vi "Set Property.vi"(10 "Ctl Ref":refnum<vi>, 11 "FontUIP In":refnum<class "FontUIP.lvclass">) -> (0 "Error Out":errorcluster, 3 "FontUIP Out":refnum<class "FontUIP.lvclass">)   [LabVIEW 2016, in "FontUIP.lvclass"]
doc: "Overwrite this abstract method to implement child behavior for applying UIP private data into the VI Server Control property."
uses:
  FontUIP.lvclass
  FontUIP.lvclass/FontUIP.ctl
  <vilib>/Utility/miscctls.llb/LVRowAndColumnTypeDef.ctl
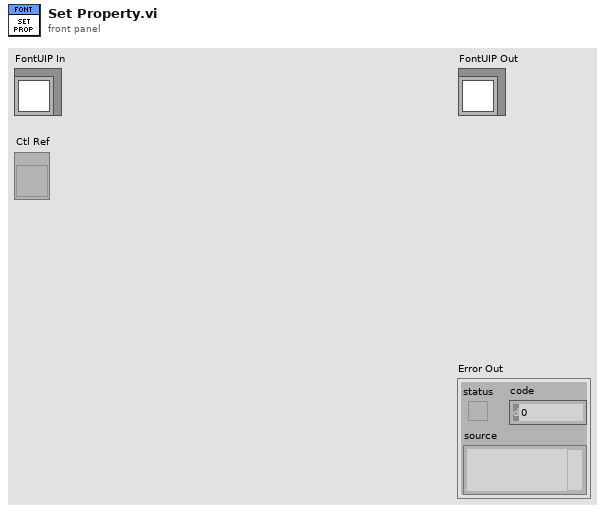
[diagram p1: front panel]
types:
  T1 = typedef "LVFontTypeDef.ctl" = cluster{"Font Name":string, "Size":u16, "Bold":bool, "Italic":bool, "Underline":bool, "Strikeout":bool, "Color":u32}
  T2 = typedef "LVRowAndColumnTypeDef.ctl" = cluster{"Row":i32, "Column":i32}
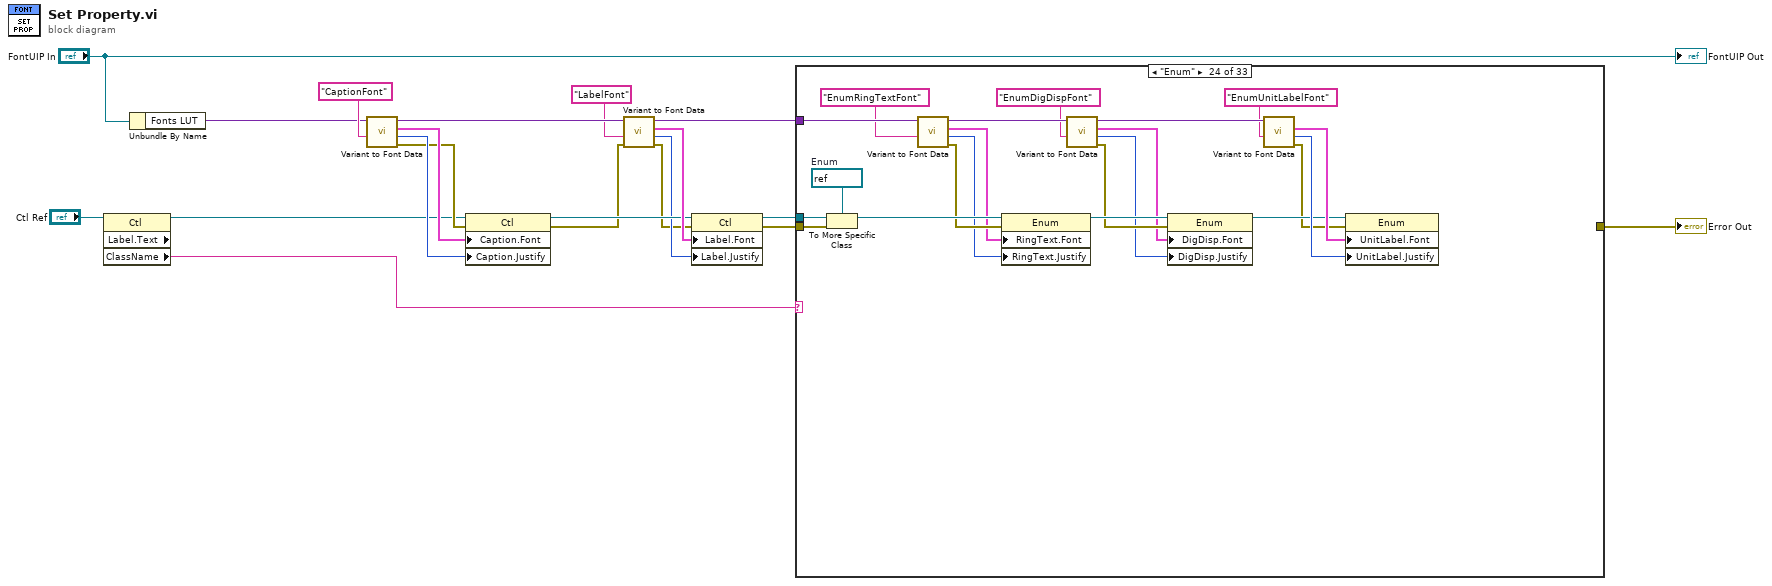
[diagram p0: block diagram]
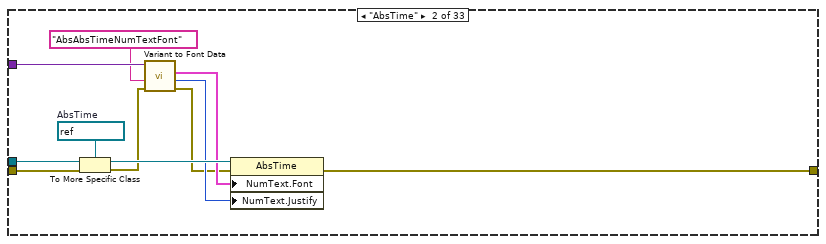
[diagram p3: hidden frame]
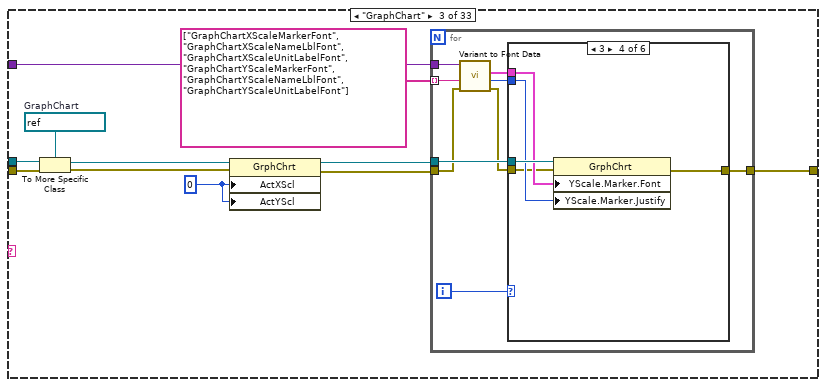
[diagram p4: hidden frame]
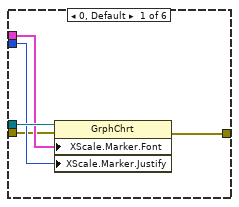
[diagram p5: hidden frame]
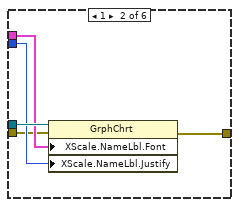
[diagram p6: hidden frame]
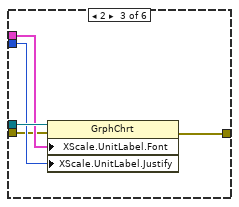
[diagram p7: hidden frame]
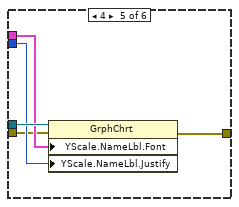
[diagram p8: hidden frame]
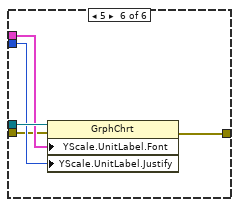
[diagram p9: hidden frame]
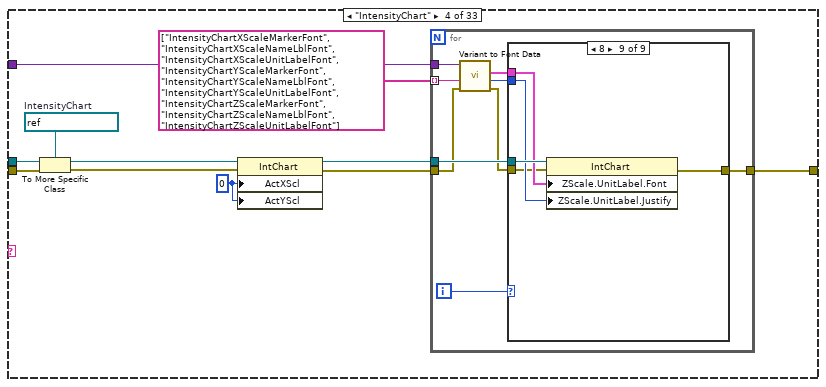
[diagram p10: hidden frame]
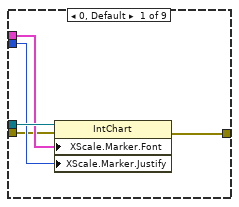
[diagram p11: hidden frame]
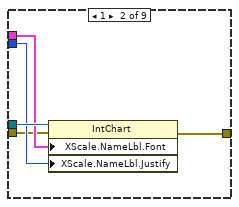
[diagram p12: hidden frame]
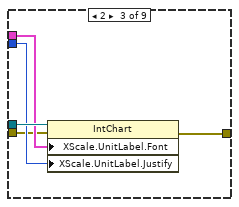
[diagram p13: hidden frame]
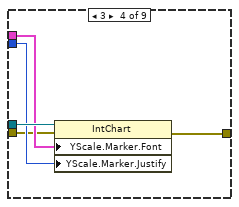
[diagram p14: hidden frame]
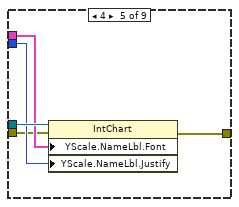
[diagram p15: hidden frame]
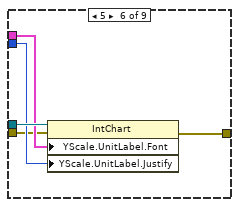
[diagram p16: hidden frame]
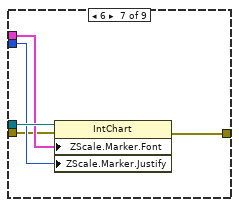
[diagram p17: hidden frame]
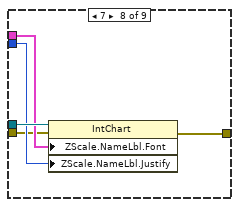
[diagram p18: hidden frame]
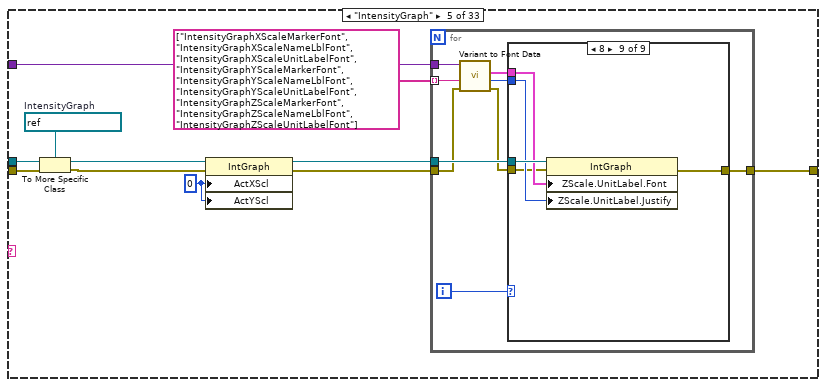
[diagram p19: hidden frame]
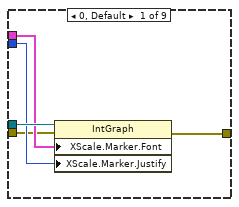
[diagram p20: hidden frame]
diagram:
  n1 = property class="Ctl" props=["Label", "Text", "ClassName"](reference="Ctl Ref") -> (reference out=w6:refnum<vi>, "ClassName"=w2:string)  [unwired: 1 in, 2 out]
  n2 = Unbundle By Name("FontUIP In") -> ("Fonts LUT"=w3:variant)
  n3 = call "Variant to Font Data.vi"("Font Key Name"="CaptionFont", "Fonts LUT in"=w3) -> ("error out"=w11:errorcluster, "Justification"=w13:enum16{"Left", "Center", "Right"}, "Font"=w12:T1, "Fonts LUT out"=w18:variant)  [unwired: 6 in]
  n4 = property class="Ctl"(reference=w6, error in=w11, "Caption.Font"=w12, "Caption.Justify"=w13) -> (reference out=w16:refnum<vi>, error out=w10:errorcluster)
  n5 = call "Variant to Font Data.vi"("error in"=w10, "Font Key Name"="LabelFont", "Fonts LUT in"=w18) -> ("error out"=w8:errorcluster, "Justification"=w9:enum16{"Left", "Center", "Right"}, "Font"=w17:T1, "Fonts LUT out"=w7:variant)  [unwired: 5 in]
  n6 = property class="Ctl"(reference=w16, error in=w8, "Label.Font"=w17, "Label.Justify"=w9) -> (reference out=w5:refnum<vi>, error out=w4:errorcluster)
  n7 = case shown="\"Enum\"" w2 {
    tunnel: w5 -> [_ w32 w42 w92 w157 w222 w272 w322 w372 w422 w473 w484 w495 w506 w517 w528 w540 w551 w563 w574 w595 w610 w631 w652 w673 w684 w701 w718 w729 w740 w751 w763 w775]
    tunnel: w7 -> [_ w27 w43 w93 w158 w223 w273 w323 w373 w423 w468 w479 w490 w501 w512 w523 w534 w546 w557 w569 w592 w607 w628 w649 w670 w679 w698 w715 w725 w735 w746 w757 w770]
    tunnel: w4 -> [w21 w31 w41 w91 w156 w221 w271 w321 w371 w421 w472 w483 w494 w505 w516 w527 w539 w550 w562 w573 w594 w609 w630 w651 w672 w683 w700 w717 w728 w739 w750 w762 w774]
    tunnel: [w21 w28 w38 w89 w153 w218 w268 w318 w368 w418 w469 w480 w491 w502 w513 w524 w535 w547 w559 w570 _ _ _ _ _ w680 _ _ w719 w736 w747 w759 w771] -> w1
    frame Default {
    }
    frame "AbsTime" {
      w29 = refnum<vi> refnum  # AbsTime
      n8 = To More Specific Class(target class=w29, reference=w32, error in=w31) -> (specific class reference=w30:refnum<vi>, error out=w23:errorcluster)
      n9 = call "Variant to Font Data.vi"("error in"=w23, "Font Key Name"="AbsAbsTimeNumTextFont", "Fonts LUT in"=w27) -> ("error out"=w22:errorcluster, "Justification"=w24:enum16{"Left", "Center", "Right"}, "Font"=w25:T1)  [unwired: 5 in, 1 out]
      n10 = property class="AbsTime"(reference=w30, error in=w22, "NumText.Font"=w25, "NumText.Justify"=w24) -> (error out=w28:errorcluster)  [unwired: 1 out]
    }
    frame "GraphChart" {
      w33 = 0 ("Active X Scale")
      w40 = refnum<vi> refnum  # GraphChart
      n11 = To More Specific Class(target class=w40, reference=w42, error in=w41) -> (specific class reference=w37:refnum<vi>, error out=w36:errorcluster)
      n12 = property class="GrphChrt"(reference=w37, error in=w36, "ActXScl"=w33, "ActYScl"=w33) -> (reference out=w35:refnum<vi>, error out=w34:errorcluster)
      n13 = for {
        tunnel: string[] ["GraphChartXScaleMarkerFont", "GraphChartXScaleNameLblFont", "GraphChartXScaleUnitLabelFont", "GraphChartYScaleMarkerFont", "GraphChartYScaleNameLblFont", "GraphChartYScaleUnitLabelFont"] -> [w51] mode=indexing
        tunnel: w43 -> [w52]
        tunnel: w35 -> [w47]
        tunnel: w34 -> [w46]
        tunnel: [w44] -> w38
        i -> [w50]
        n14 = call "Variant to Font Data.vi"("error in"=w46, "Font Key Name"=w51, "Fonts LUT in"=w52) -> ("error out"=w45:errorcluster, "Justification"=w48:enum16{"Left", "Center", "Right"}, "Font"=w49:T1)  [unwired: 5 in, 1 out]
        n15 = case shown="3" w50 {
          tunnel: w49 -> [w56 w61 w66 w71 w76 w81]
          tunnel: w48 -> [w55 w60 w65 w70 w75 w80]
          tunnel: w47 -> [w57 w62 w67 w72 w77 w82]
          tunnel: w45 -> [w54 w59 w64 w69 w74 w79]
          tunnel: [w53 w58 w63 w68 w73 w78] -> w44
          frame 0, Default {
            n16 = property class="GrphChrt"(reference=w57, error in=w54, "XScale.Marker.Font"=w56, "XScale.Marker.Justify"=w55) -> (error out=w53:errorcluster)  [unwired: 1 out]
          }
          frame 1 {
            n17 = property class="GrphChrt"(reference=w62, error in=w59, "XScale.NameLbl.Font"=w61, "XScale.NameLbl.Justify"=w60) -> (error out=w58:errorcluster)  [unwired: 1 out]
          }
          frame 2 {
            n18 = property class="GrphChrt"(reference=w67, error in=w64, "XScale.UnitLabel.Font"=w66, "XScale.UnitLabel.Justify"=w65) -> (error out=w63:errorcluster)  [unwired: 1 out]
          }
          frame 3 {
            n19 = property class="GrphChrt"(reference=w72, error in=w69, "YScale.Marker.Font"=w71, "YScale.Marker.Justify"=w70) -> (error out=w68:errorcluster)  [unwired: 1 out]
          }
          frame 4 {
            n20 = property class="GrphChrt"(reference=w77, error in=w74, "YScale.NameLbl.Font"=w76, "YScale.NameLbl.Justify"=w75) -> (error out=w73:errorcluster)  [unwired: 1 out]
          }
          frame 5 {
            n21 = property class="GrphChrt"(reference=w82, error in=w79, "YScale.UnitLabel.Font"=w81, "YScale.UnitLabel.Justify"=w80) -> (error out=w78:errorcluster)  [unwired: 1 out]
          }
        }
      }
    }
    frame "IntensityChart" {
      w83 = 0 ("Active X Scale")
      w90 = refnum<vi> refnum  # IntensityChart
      n22 = To More Specific Class(target class=w90, reference=w92, error in=w91) -> (specific class reference=w87:refnum<vi>, error out=w86:errorcluster)
      n23 = property class="IntChart"(reference=w87, error in=w86, "ActXScl"=w83, "ActYScl"=w83) -> (reference out=w85:refnum<vi>, error out=w84:errorcluster)
      n24 = for {
        tunnel: string[] ["IntensityChartXScaleMarkerFont", "IntensityChartXScaleNameLblFont", "IntensityChartXScaleUnitLabelFont", "IntensityChartYScaleMarkerFont", "IntensityChartYScaleNameLblFont", "IntensityChartYScaleUnitLabelFont", "IntensityChartZScaleMarkerFont", "IntensityChartZScaleNameLblFont", "IntensityChartZScaleUnitLabelFont"] -> [w101] mode=indexing
        tunnel: w93 -> [w102]
        tunnel: w85 -> [w97]
        tunnel: w84 -> [w96]
        tunnel: [w94] -> w89
        i -> [w100]
        n25 = call "Variant to Font Data.vi"("error in"=w96, "Font Key Name"=w101, "Fonts LUT in"=w102) -> ("error out"=w95:errorcluster, "Justification"=w98:enum16{"Left", "Center", "Right"}, "Font"=w99:T1)  [unwired: 5 in, 1 out]
        n26 = case shown="8" w100 {
          tunnel: w99 -> [w106 w111 w116 w121 w126 w131 w136 w141 w146]
          tunnel: w98 -> [w105 w110 w115 w120 w125 w130 w135 w140 w145]
          tunnel: w97 -> [w107 w112 w117 w122 w127 w132 w137 w142 w147]
          tunnel: w95 -> [w104 w109 w114 w119 w124 w129 w134 w139 w144]
          tunnel: [w103 w108 w113 w118 w123 w128 w133 w138 w143] -> w94
          frame 0, Default {
            n27 = property class="IntChart"(reference=w107, error in=w104, "XScale.Marker.Font"=w106, "XScale.Marker.Justify"=w105) -> (error out=w103:errorcluster)  [unwired: 1 out]
          }
          frame 1 {
            n28 = property class="IntChart"(reference=w112, error in=w109, "XScale.NameLbl.Font"=w111, "XScale.NameLbl.Justify"=w110) -> (error out=w108:errorcluster)  [unwired: 1 out]
          }
          frame 2 {
            n29 = property class="IntChart"(reference=w117, error in=w114, "XScale.UnitLabel.Font"=w116, "XScale.UnitLabel.Justify"=w115) -> (error out=w113:errorcluster)  [unwired: 1 out]
          }
          frame 3 {
            n30 = property class="IntChart"(reference=w122, error in=w119, "YScale.Marker.Font"=w121, "YScale.Marker.Justify"=w120) -> (error out=w118:errorcluster)  [unwired: 1 out]
          }
          frame 4 {
            n31 = property class="IntChart"(reference=w127, error in=w124, "YScale.NameLbl.Font"=w126, "YScale.NameLbl.Justify"=w125) -> (error out=w123:errorcluster)  [unwired: 1 out]
          }
          frame 5 {
            n32 = property class="IntChart"(reference=w132, error in=w129, "YScale.UnitLabel.Font"=w131, "YScale.UnitLabel.Justify"=w130) -> (error out=w128:errorcluster)  [unwired: 1 out]
          }
          frame 6 {
            n33 = property class="IntChart"(reference=w137, error in=w134, "ZScale.Marker.Font"=w136, "ZScale.Marker.Justify"=w135) -> (error out=w133:errorcluster)  [unwired: 1 out]
          }
          frame 7 {
            n34 = property class="IntChart"(reference=w142, error in=w139, "ZScale.NameLbl.Font"=w141, "ZScale.NameLbl.Justify"=w140) -> (error out=w138:errorcluster)  [unwired: 1 out]
          }
          frame 8 {
            n35 = property class="IntChart"(reference=w147, error in=w144, "ZScale.UnitLabel.Font"=w146, "ZScale.UnitLabel.Justify"=w145) -> (error out=w143:errorcluster)  [unwired: 1 out]
          }
        }
      }
    }
    frame "IntensityGraph" {
      w148 = 0 ("Active X Scale")
      w155 = refnum<vi> refnum  # IntensityGraph
      n36 = To More Specific Class(target class=w155, reference=w157, error in=w156) -> (specific class reference=w154:refnum<vi>, error out=w150:errorcluster)
      n37 = property class="IntGraph"(reference=w154, error in=w150, "ActXScl"=w148, "ActYScl"=w148) -> (reference out=w151:refnum<vi>, error out=w149:errorcluster)
      n38 = for {
        tunnel: string[] ["IntensityGraphXScaleMarkerFont", "IntensityGraphXScaleNameLblFont", "IntensityGraphXScaleUnitLabelFont", "IntensityGraphYScaleMarkerFont", "IntensityGraphYScaleNameLblFont", "IntensityGraphYScaleUnitLabelFont", "IntensityGraphZScaleMarkerFont", "IntensityGraphZScaleNameLblFont", "IntensityGraphZScaleUnitLabelFont"] -> [w166] mode=indexing
        tunnel: w158 -> [w167]
        tunnel: w151 -> [w162]
        tunnel: w149 -> [w161]
        tunnel: [w159] -> w153
        i -> [w165]
        n39 = call "Variant to Font Data.vi"("error in"=w161, "Font Key Name"=w166, "Fonts LUT in"=w167) -> ("error out"=w160:errorcluster, "Justification"=w163:enum16{"Left", "Center", "Right"}, "Font"=w164:T1)  [unwired: 5 in, 1 out]
        n40 = case shown="8" w165 {
          tunnel: w164 -> [w171 w176 w181 w186 w191 w196 w201 w206 w211]
          tunnel: w163 -> [w170 w175 w180 w185 w190 w195 w200 w205 w210]
          tunnel: w162 -> [w172 w177 w182 w187 w192 w197 w202 w207 w212]
          tunnel: w160 -> [w169 w174 w179 w184 w189 w194 w199 w204 w209]
          tunnel: [w168 w173 w178 w183 w188 w193 w198 w203 w208] -> w159
          frame 0, Default {
            n41 = property class="IntGraph"(reference=w172, error in=w169, "XScale.Marker.Font"=w171, "XScale.Marker.Justify"=w170) -> (error out=w168:errorcluster)  [unwired: 1 out]
          }
          frame 1 {
            n42 = property class="IntGraph"(reference=w177, error in=w174, "XScale.NameLbl.Font"=w176, "XScale.NameLbl.Justify"=w175) -> (error out=w173:errorcluster)  [unwired: 1 out]
          }
          frame 2 {
            n43 = property class="IntGraph"(reference=w182, error in=w179, "XScale.UnitLabel.Font"=w181, "XScale.UnitLabel.Justify"=w180) -> (error out=w178:errorcluster)  [unwired: 1 out]
          }
          frame 3 {
            n44 = property class="IntGraph"(reference=w187, error in=w184, "YScale.Marker.Font"=w186, "YScale.Marker.Justify"=w185) -> (error out=w183:errorcluster)  [unwired: 1 out]
          }
          frame 4 {
            n45 = property class="IntGraph"(reference=w192, error in=w189, "YScale.NameLbl.Font"=w191, "YScale.NameLbl.Justify"=w190) -> (error out=w188:errorcluster)  [unwired: 1 out]
          }
          frame 5 {
            n46 = property class="IntGraph"(reference=w197, error in=w194, "YScale.UnitLabel.Font"=w196, "YScale.UnitLabel.Justify"=w195) -> (error out=w193:errorcluster)  [unwired: 1 out]
          }
          frame 6 {
            n47 = property class="IntGraph"(reference=w202, error in=w199, "ZScale.Marker.Font"=w201, "ZScale.Marker.Justify"=w200) -> (error out=w198:errorcluster)  [unwired: 1 out]
          }
          frame 7 {
            n48 = property class="IntGraph"(reference=w207, error in=w204, "ZScale.NameLbl.Font"=w206, "ZScale.NameLbl.Justify"=w205) -> (error out=w203:errorcluster)  [unwired: 1 out]
          }
          frame 8 {
            n49 = property class="IntGraph"(reference=w212, error in=w209, "ZScale.UnitLabel.Font"=w211, "ZScale.UnitLabel.Justify"=w210) -> (error out=w208:errorcluster)  [unwired: 1 out]
          }
        }
      }
    }
    frame "MixedSignalGraph" {
      w213 = 0 ("Active X Scale")
      w220 = refnum<vi> refnum  # MixedSignalGraph
      n50 = To More Specific Class(target class=w220, reference=w222, error in=w221) -> (specific class reference=w219:refnum<vi>, error out=w215:errorcluster)
      n51 = property class="MixedGraph"(reference=w219, error in=w215, "ActXScl"=w213, "ActYScl"=w213) -> (reference out=w216:refnum<vi>, error out=w214:errorcluster)
      n52 = for {
        tunnel: string[] ["MixedSignalGraphXScaleMarkerFont", "MixedSignalGraphXScaleNameLblFont", "MixedSignalGraphXScaleUnitLabelFont", "MixedSignalGraphYScaleMarkerFont", "MixedSignalGraphYScaleNameLblFont", "MixedSignalGraphYScaleUnitLabelFont"] -> [w231] mode=indexing
        tunnel: w223 -> [w232]
        tunnel: w216 -> [w227]
        tunnel: w214 -> [w226]
        tunnel: [w224] -> w218
        i -> [w230]
        n53 = call "Variant to Font Data.vi"("error in"=w226, "Font Key Name"=w231, "Fonts LUT in"=w232) -> ("error out"=w225:errorcluster, "Justification"=w228:enum16{"Left", "Center", "Right"}, "Font"=w229:T1)  [unwired: 5 in, 1 out]
        n54 = case shown="0, Default" w230 {
          tunnel: w229 -> [w236 w241 w246 w251 w256 w261]
          tunnel: w228 -> [w235 w240 w245 w250 w255 w260]
          tunnel: w227 -> [w237 w242 w247 w252 w257 w262]
          tunnel: w225 -> [w234 w239 w244 w249 w254 w259]
          tunnel: [w233 w238 w243 w248 w253 w258] -> w224
          frame 0, Default {
            n55 = property class="MixedGraph"(reference=w237, error in=w234, "XScale.Marker.Font"=w236, "XScale.Marker.Justify"=w235) -> (error out=w233:errorcluster)  [unwired: 1 out]
          }
          frame 1 {
            n56 = property class="MixedGraph"(reference=w242, error in=w239, "XScale.NameLbl.Font"=w241, "XScale.NameLbl.Justify"=w240) -> (error out=w238:errorcluster)  [unwired: 1 out]
          }
          frame 2 {
            n57 = property class="MixedGraph"(reference=w247, error in=w244, "XScale.UnitLabel.Font"=w246, "XScale.UnitLabel.Justify"=w245) -> (error out=w243:errorcluster)  [unwired: 1 out]
          }
          frame 3 {
            n58 = property class="MixedGraph"(reference=w252, error in=w249, "YScale.Marker.Font"=w251, "YScale.Marker.Justify"=w250) -> (error out=w248:errorcluster)  [unwired: 1 out]
          }
          frame 4 {
            n59 = property class="MixedGraph"(reference=w257, error in=w254, "YScale.NameLbl.Font"=w256, "YScale.NameLbl.Justify"=w255) -> (error out=w253:errorcluster)  [unwired: 1 out]
          }
          frame 5 {
            n60 = property class="MixedGraph"(reference=w262, error in=w259, "YScale.UnitLabel.Font"=w261, "YScale.UnitLabel.Justify"=w260) -> (error out=w258:errorcluster)  [unwired: 1 out]
          }
        }
      }
    }
    frame "WaveformChart" {
      w263 = 0 ("Active X Scale")
      w270 = refnum<vi> refnum  # WaveformChart
      n61 = To More Specific Class(target class=w270, reference=w272, error in=w271) -> (specific class reference=w269:refnum<vi>, error out=w265:errorcluster)
      n62 = property class="WFChart"(reference=w269, error in=w265, "ActXScl"=w263, "ActYScl"=w263) -> (reference out=w266:refnum<vi>, error out=w264:errorcluster)
      n63 = for {
        tunnel: string[] ["WaveformChartXScaleMarkerFont", "WaveformChartXScaleNameLblFont", "WaveformChartXScaleUnitLabelFont", "WaveformChartYScaleMarkerFont", "WaveformChartYScaleNameLblFont", "WaveformChartYScaleUnitLabelFont"] -> [w281] mode=indexing
        tunnel: w273 -> [w282]
        tunnel: w266 -> [w277]
        tunnel: w264 -> [w276]
        tunnel: [w274] -> w268
        i -> [w280]
        n64 = call "Variant to Font Data.vi"("error in"=w276, "Font Key Name"=w281, "Fonts LUT in"=w282) -> ("error out"=w275:errorcluster, "Justification"=w278:enum16{"Left", "Center", "Right"}, "Font"=w279:T1)  [unwired: 5 in, 1 out]
        n65 = case shown="5" w280 {
          tunnel: w279 -> [w286 w291 w296 w301 w306 w311]
          tunnel: w278 -> [w285 w290 w295 w300 w305 w310]
          tunnel: w277 -> [w287 w292 w297 w302 w307 w312]
          tunnel: w275 -> [w284 w289 w294 w299 w304 w309]
          tunnel: [w283 w288 w293 w298 w303 w308] -> w274
          frame 0, Default {
            n66 = property class="WFChart"(reference=w287, error in=w284, "XScale.Marker.Font"=w286, "XScale.Marker.Justify"=w285) -> (error out=w283:errorcluster)  [unwired: 1 out]
          }
          frame 1 {
            n67 = property class="WFChart"(reference=w292, error in=w289, "XScale.NameLbl.Font"=w291, "XScale.NameLbl.Justify"=w290) -> (error out=w288:errorcluster)  [unwired: 1 out]
          }
          frame 2 {
            n68 = property class="WFChart"(reference=w297, error in=w294, "XScale.UnitLabel.Font"=w296, "XScale.UnitLabel.Justify"=w295) -> (error out=w293:errorcluster)  [unwired: 1 out]
          }
          frame 3 {
            n69 = property class="WFChart"(reference=w302, error in=w299, "YScale.Marker.Font"=w301, "YScale.Marker.Justify"=w300) -> (error out=w298:errorcluster)  [unwired: 1 out]
          }
          frame 4 {
            n70 = property class="WFChart"(reference=w307, error in=w304, "YScale.NameLbl.Font"=w306, "YScale.NameLbl.Justify"=w305) -> (error out=w303:errorcluster)  [unwired: 1 out]
          }
          frame 5 {
            n71 = property class="WFChart"(reference=w312, error in=w309, "YScale.UnitLabel.Font"=w311, "YScale.UnitLabel.Justify"=w310) -> (error out=w308:errorcluster)  [unwired: 1 out]
          }
        }
      }
    }
    frame "WaveformGraph" {
      w313 = 0 ("Active X Scale")
      w320 = refnum<vi> refnum  # WaveformGraph
      n72 = To More Specific Class(target class=w320, reference=w322, error in=w321) -> (specific class reference=w319:refnum<vi>, error out=w315:errorcluster)
      n73 = property class="WFGraph"(reference=w319, error in=w315, "ActXScl"=w313, "ActYScl"=w313) -> (reference out=w316:refnum<vi>, error out=w314:errorcluster)
      n74 = for {
        tunnel: string[] ["WaveformGraphXScaleMarkerFont", "WaveformGraphXScaleNameLblFont", "WaveformGraphXScaleUnitLabelFont", "WaveformGraphYScaleMarkerFont", "WaveformGraphYScaleNameLblFont", "WaveformGraphYScaleUnitLabelFont"] -> [w331] mode=indexing
        tunnel: w323 -> [w332]
        tunnel: w316 -> [w327]
        tunnel: w314 -> [w326]
        tunnel: [w324] -> w318
        i -> [w330]
        n75 = call "Variant to Font Data.vi"("error in"=w326, "Font Key Name"=w331, "Fonts LUT in"=w332) -> ("error out"=w325:errorcluster, "Justification"=w328:enum16{"Left", "Center", "Right"}, "Font"=w329:T1)  [unwired: 5 in, 1 out]
        n76 = case shown="4" w330 {
          tunnel: w329 -> [w336 w341 w346 w351 w356 w361]
          tunnel: w328 -> [w335 w340 w345 w350 w355 w360]
          tunnel: w327 -> [w337 w342 w347 w352 w357 w362]
          tunnel: w325 -> [w334 w339 w344 w349 w354 w359]
          tunnel: [w333 w338 w343 w348 w353 w358] -> w324
          frame 0, Default {
            n77 = property class="WFGraph"(reference=w337, error in=w334, "XScale.Marker.Font"=w336, "XScale.Marker.Justify"=w335) -> (error out=w333:errorcluster)  [unwired: 1 out]
          }
          frame 1 {
            n78 = property class="WFGraph"(reference=w342, error in=w339, "XScale.NameLbl.Font"=w341, "XScale.NameLbl.Justify"=w340) -> (error out=w338:errorcluster)  [unwired: 1 out]
          }
          frame 2 {
            n79 = property class="WFGraph"(reference=w347, error in=w344, "XScale.UnitLabel.Font"=w346, "XScale.UnitLabel.Justify"=w345) -> (error out=w343:errorcluster)  [unwired: 1 out]
          }
          frame 3 {
            n80 = property class="WFGraph"(reference=w352, error in=w349, "YScale.Marker.Font"=w351, "YScale.Marker.Justify"=w350) -> (error out=w348:errorcluster)  [unwired: 1 out]
          }
          frame 4 {
            n81 = property class="WFGraph"(reference=w357, error in=w354, "YScale.NameLbl.Font"=w356, "YScale.NameLbl.Justify"=w355) -> (error out=w353:errorcluster)  [unwired: 1 out]
          }
          frame 5 {
            n82 = property class="WFGraph"(reference=w362, error in=w359, "YScale.UnitLabel.Font"=w361, "YScale.UnitLabel.Justify"=w360) -> (error out=w358:errorcluster)  [unwired: 1 out]
          }
        }
      }
    }
    frame "DigitalGraph" {
      w363 = 0 ("Active X Scale")
      w370 = refnum<vi> refnum  # DigitalGraph
      n83 = To More Specific Class(target class=w370, reference=w372, error in=w371) -> (specific class reference=w369:refnum<vi>, error out=w365:errorcluster)
      n84 = property class="DigitalGraph"(reference=w369, error in=w365, "ActXScl"=w363, "ActYScl"=w363) -> (reference out=w366:refnum<vi>, error out=w364:errorcluster)
      n85 = for {
        tunnel: string[] ["DigitalGraphXScaleMarkerFont", "DigitalGraphXScaleNameLblFont", "DigitalGraphXScaleUnitLabelFont", "DigitalGraphYScaleMarkerFont", "DigitalGraphYScaleNameLblFont", "DigitalGraphYScaleUnitLabelFont"] -> [w381] mode=indexing
        tunnel: w373 -> [w382]
        tunnel: w366 -> [w377]
        tunnel: w364 -> [w376]
        tunnel: [w374] -> w368
        i -> [w380]
        n86 = call "Variant to Font Data.vi"("error in"=w376, "Font Key Name"=w381, "Fonts LUT in"=w382) -> ("error out"=w375:errorcluster, "Justification"=w378:enum16{"Left", "Center", "Right"}, "Font"=w379:T1)  [unwired: 5 in, 1 out]
        n87 = case shown="1" w380 {
          tunnel: w379 -> [w386 w391 w396 w401 w406 w411]
          tunnel: w378 -> [w385 w390 w395 w400 w405 w410]
          tunnel: w377 -> [w387 w392 w397 w402 w407 w412]
          tunnel: w375 -> [w384 w389 w394 w399 w404 w409]
          tunnel: [w383 w388 w393 w398 w403 w408] -> w374
          frame 0, Default {
            n88 = property class="DigitalGraph"(reference=w387, error in=w384, "XScale.Marker.Font"=w386, "XScale.Marker.Justify"=w385) -> (error out=w383:errorcluster)  [unwired: 1 out]
          }
          frame 1 {
            n89 = property class="DigitalGraph"(reference=w392, error in=w389, "XScale.NameLbl.Font"=w391, "XScale.NameLbl.Justify"=w390) -> (error out=w388:errorcluster)  [unwired: 1 out]
          }
          frame 2 {
            n90 = property class="DigitalGraph"(reference=w397, error in=w394, "XScale.UnitLabel.Font"=w396, "XScale.UnitLabel.Justify"=w395) -> (error out=w393:errorcluster)  [unwired: 1 out]
          }
          frame 3 {
            n91 = property class="DigitalGraph"(reference=w402, error in=w399, "YScale.Marker.Font"=w401, "YScale.Marker.Justify"=w400) -> (error out=w398:errorcluster)  [unwired: 1 out]
          }
          frame 4 {
            n92 = property class="DigitalGraph"(reference=w407, error in=w404, "YScale.NameLbl.Font"=w406, "YScale.NameLbl.Justify"=w405) -> (error out=w403:errorcluster)  [unwired: 1 out]
          }
          frame 5 {
            n93 = property class="DigitalGraph"(reference=w412, error in=w409, "YScale.UnitLabel.Font"=w411, "YScale.UnitLabel.Justify"=w410) -> (error out=w408:errorcluster)  [unwired: 1 out]
          }
        }
      }
    }
    frame "XYGraph" {
      w413 = 0 ("Active X Scale")
      w420 = refnum<vi> refnum  # XYGraph
      n94 = To More Specific Class(target class=w420, reference=w422, error in=w421) -> (specific class reference=w419:refnum<vi>, error out=w415:errorcluster)
      n95 = property class="XYGraph"(reference=w419, error in=w415, "ActXScl"=w413, "ActYScl"=w413) -> (reference out=w416:refnum<vi>, error out=w414:errorcluster)
      n96 = for {
        tunnel: string[] ["XYGraphXScaleMarkerFont", "XYGraphXScaleNameLblFont", "XYGraphXScaleUnitLabelFont", "XYGraphYScaleMarkerFont", "XYGraphYScaleNameLblFont", "XYGraphYScaleUnitLabelFont"] -> [w431] mode=indexing
        tunnel: w423 -> [w432]
        tunnel: w416 -> [w427]
        tunnel: w414 -> [w426]
        tunnel: [w424] -> w418
        i -> [w430]
        n97 = call "Variant to Font Data.vi"("error in"=w426, "Font Key Name"=w431, "Fonts LUT in"=w432) -> ("error out"=w425:errorcluster, "Justification"=w428:enum16{"Left", "Center", "Right"}, "Font"=w429:T1)  [unwired: 5 in, 1 out]
        n98 = case shown="1" w430 {
          tunnel: w429 -> [w436 w441 w446 w451 w456 w461]
          tunnel: w428 -> [w435 w440 w445 w450 w455 w460]
          tunnel: w427 -> [w437 w442 w447 w452 w457 w462]
          tunnel: w425 -> [w434 w439 w444 w449 w454 w459]
          tunnel: [w433 w438 w443 w448 w453 w458] -> w424
          frame 0, Default {
            n99 = property class="XYGraph"(reference=w437, error in=w434, "XScale.Marker.Font"=w436, "XScale.Marker.Justify"=w435) -> (error out=w433:errorcluster)  [unwired: 1 out]
          }
          frame 1 {
            n100 = property class="XYGraph"(reference=w442, error in=w439, "XScale.NameLbl.Font"=w441, "XScale.NameLbl.Justify"=w440) -> (error out=w438:errorcluster)  [unwired: 1 out]
          }
          frame 2 {
            n101 = property class="XYGraph"(reference=w447, error in=w444, "XScale.UnitLabel.Font"=w446, "XScale.UnitLabel.Justify"=w445) -> (error out=w443:errorcluster)  [unwired: 1 out]
          }
          frame 3 {
            n102 = property class="XYGraph"(reference=w452, error in=w449, "YScale.Marker.Font"=w451, "YScale.Marker.Justify"=w450) -> (error out=w448:errorcluster)  [unwired: 1 out]
          }
          frame 4 {
            n103 = property class="XYGraph"(reference=w457, error in=w454, "YScale.NameLbl.Font"=w456, "YScale.NameLbl.Justify"=w455) -> (error out=w453:errorcluster)  [unwired: 1 out]
          }
          frame 5 {
            n104 = property class="XYGraph"(reference=w462, error in=w459, "YScale.UnitLabel.Font"=w461, "YScale.UnitLabel.Justify"=w460) -> (error out=w458:errorcluster)  [unwired: 1 out]
          }
        }
      }
    }
    frame "Boolean" {
      w470 = refnum<vi> refnum  # Boolean
      n105 = To More Specific Class(target class=w470, reference=w473, error in=w472) -> (specific class reference=w471:refnum<vi>, error out=w467:errorcluster)
      n106 = call "Variant to Font Data.vi"("error in"=w467, "Font Key Name"="BooleanBoolTextFont", "Fonts LUT in"=w468) -> ("error out"=w466:errorcluster, "Justification"=w464:enum16{"Left", "Center", "Right"}, "Font"=w465:T1)  [unwired: 5 in, 1 out]
      n107 = property class="Bool"(reference=w471, error in=w466, "BoolText.Font"=w465, "BoolText.Justify"=w464) -> (error out=w469:errorcluster)  [unwired: 1 out]
    }
    frame "IOName" {
      w481 = refnum<vi> refnum  # IOName
      n108 = To More Specific Class(target class=w481, reference=w484, error in=w483) -> (specific class reference=w482:refnum<vi>, error out=w478:errorcluster)
      n109 = call "Variant to Font Data.vi"("error in"=w478, "Font Key Name"="IONameTextFont", "Fonts LUT in"=w479) -> ("error out"=w477:errorcluster, "Justification"=w475:enum16{"Left", "Center", "Right"}, "Font"=w476:T1)  [unwired: 5 in, 1 out]
      n110 = property class="IOName"(reference=w482, error in=w477, "Text.Font"=w476, "Text.Justify"=w475) -> (error out=w480:errorcluster)  [unwired: 1 out]
    }
    frame "DAQChannelName" {
      w492 = refnum<vi> refnum  # DAQChannelName
      n111 = To More Specific Class(target class=w492, reference=w495, error in=w494) -> (specific class reference=w493:refnum<vi>, error out=w489:errorcluster)
      n112 = call "Variant to Font Data.vi"("error in"=w489, "Font Key Name"="DAQChannelNameTextFont", "Fonts LUT in"=w490) -> ("error out"=w488:errorcluster, "Justification"=w485:enum16{"Left", "Center", "Right"}, "Font"=w486:T1)  [unwired: 5 in, 1 out]
      n113 = property class="DAQName"(reference=w493, error in=w488, "Text.Font"=w486, "Text.Justify"=w485) -> (error out=w491:errorcluster)  [unwired: 1 out]
    }
    frame "DAQmxName" {
      w503 = refnum<vi> refnum  # DAQmxName
      n114 = To More Specific Class(target class=w503, reference=w506, error in=w505) -> (specific class reference=w504:refnum<vi>, error out=w500:errorcluster)
      n115 = call "Variant to Font Data.vi"("error in"=w500, "Font Key Name"="DAQmxNameTextFont", "Fonts LUT in"=w501) -> ("error out"=w499:errorcluster, "Justification"=w497:enum16{"Left", "Center", "Right"}, "Font"=w496:T1)  [unwired: 5 in, 1 out]
      n116 = property class="DAQmxName"(reference=w504, error in=w499, "Text.Font"=w496, "Text.Justify"=w497) -> (error out=w502:errorcluster)  [unwired: 1 out]
    }
    frame "IVILogicalName" {
      w514 = refnum<vi> refnum  # IVILogicalName
      n117 = To More Specific Class(target class=w514, reference=w517, error in=w516) -> (specific class reference=w515:refnum<vi>, error out=w510:errorcluster)
      n118 = call "Variant to Font Data.vi"("error in"=w510, "Font Key Name"="IVILogicalNameTextFont", "Fonts LUT in"=w512) -> ("error out"=w509:errorcluster, "Justification"=w507:enum16{"Left", "Center", "Right"}, "Font"=w508:T1)  [unwired: 5 in, 1 out]
      n119 = property class="IVIName"(reference=w515, error in=w509, "Text.Font"=w508, "Text.Justify"=w507) -> (error out=w513:errorcluster)  [unwired: 1 out]
    }
    frame "VISAResourceName" {
      w525 = refnum<vi> refnum  # VISAResourceName
      n120 = To More Specific Class(target class=w525, reference=w528, error in=w527) -> (specific class reference=w526:refnum<vi>, error out=w522:errorcluster)
      n121 = call "Variant to Font Data.vi"("error in"=w522, "Font Key Name"="VISAResourceNameTextFont", "Fonts LUT in"=w523) -> ("error out"=w521:errorcluster, "Justification"=w519:enum16{"Left", "Center", "Right"}, "Font"=w520:T1)  [unwired: 5 in, 1 out]
      n122 = property class="VISAName"(reference=w526, error in=w521, "Text.Font"=w520, "Text.Justify"=w519) -> (error out=w524:errorcluster)  [unwired: 1 out]
    }
    frame "ListBox" {
      w537 = refnum<vi> refnum  # ListBox
      n123 = To More Specific Class(target class=w537, reference=w540, error in=w539) -> (specific class reference=w538:refnum<vi>, error out=w532:errorcluster)
      n124 = call "Variant to Font Data.vi"("error in"=w532, "Font Key Name"="ListBoxActiveRowFont", "Fonts LUT in"=w534) -> ("error out"=w531:errorcluster, "Justification"=w529:enum16{"Left", "Center", "Right"}, "Font"=w530:T1)  [unwired: 5 in, 1 out]
      n125 = property class="LstBox"(reference=w538, error in=w531, "Active Row"=-2 ("Active Row:Active Row Number"), "CellFont"=w530, "Justify"=w529) -> (error out=w535:errorcluster)  [unwired: 1 out]
    }
    frame "MixedCheckbox" {
      w548 = refnum<vi> refnum  # MixedCheckbox
      n126 = To More Specific Class(target class=w548, reference=w551, error in=w550) -> (specific class reference=w549:refnum<vi>, error out=w544:errorcluster)
      n127 = call "Variant to Font Data.vi"("error in"=w544, "Font Key Name"="MixedCheckboxTextFont", "Fonts LUT in"=w546) -> ("error out"=w543:errorcluster, "Justification"=w541:enum16{"Left", "Center", "Right"}, "Font"=w542:T1)  [unwired: 5 in, 1 out]
      n128 = property class="MixedCheckbox"(reference=w549, error in=w543, "Text.Font"=w542, "Text.Justify"=w541) -> (error out=w547:errorcluster)  [unwired: 1 out]
    }
    frame "MulticolumnListbox" {
      w560 = refnum<vi> refnum  # MulticolumnListbox
      n129 = To More Specific Class(target class=w560, reference=w563, error in=w562) -> (specific class reference=w561:refnum<vi>, error out=w555:errorcluster)
      n130 = call "Variant to Font Data.vi"("error in"=w555, "Font Key Name"="MulticolumnListboxActiveCellFont", "Fonts LUT in"=w557) -> ("error out"=w554:errorcluster, "Justification"=w552:enum16{"Left", "Center", "Right"}, "Font"=w553:T1)  [unwired: 5 in, 1 out]
      n131 = property class="MCListbox"(reference=w561, error in=w554, "ActiveCell"=T2 {"Row"=-2, "Column"=-2} ("Active Cell:Active Cell"), "CellFont"=w553, "Justify"=w552) -> (error out=w559:errorcluster)  [unwired: 1 out]
    }
    frame "Numeric" {
      w571 = refnum<vi> refnum  # Numeric
      n132 = To More Specific Class(target class=w571, reference=w574, error in=w573) -> (specific class reference=w572:refnum<vi>, error out=w568:errorcluster)
      n133 = call "Variant to Font Data.vi"("error in"=w568, "Font Key Name"="NumericUnitLabelFont", "Fonts LUT in"=w569) -> ("error out"=w567:errorcluster, "Justification"=w565:enum16{"Left", "Center", "Right"}, "Font"=w566:T1)  [unwired: 5 in, 1 out]
      n134 = property class="Num"(reference=w572, error in=w567, "UnitLabel.Font"=w566, "UnitLabel.Justify"=w565) -> (error out=w570:errorcluster)  [unwired: 1 out]
    }
    frame "ColorRamp" {
      w593 = refnum<vi> refnum  # ColorRamp
      n135 = To More Specific Class(target class=w593, reference=w595, error in=w594) -> (specific class reference=w580:refnum<vi>)  [unwired: 1 out]
      n136 = call "Variant to Font Data.vi"("Font Key Name"="ColorRampScaleMarkerFont", "Fonts LUT in"=w592) -> ("error out"=w575:errorcluster, "Justification"=w578:enum16{"Left", "Center", "Right"}, "Font"=w579:T1, "Fonts LUT out"=w591:variant)  [unwired: 6 in]
      n137 = property class="ColRmp"(reference=w580, error in=w575, "Scale.Marker.Font"=w579, "Scale.Marker.Justify"=w578) -> (reference out=w581:refnum<vi>)  [unwired: 1 out]
      n138 = call "Variant to Font Data.vi"("Font Key Name"="ColorRampDigDispFont", "Fonts LUT in"=w591) -> ("error out"=w576:errorcluster, "Justification"=w582:enum16{"Left", "Center", "Right"}, "Font"=w583:T1, "Fonts LUT out"=w590:variant)  [unwired: 6 in]
      n139 = property class="ColRmp"(reference=w581, error in=w576, "DigDisp.Font"=w583, "DigDisp.Justify"=w582) -> (reference out=w584:refnum<vi>)  [unwired: 1 out]
      n140 = call "Variant to Font Data.vi"("Font Key Name"="ColorRampUnitLabelFont", "Fonts LUT in"=w590) -> ("error out"=w577:errorcluster, "Justification"=w585:enum16{"Left", "Center", "Right"}, "Font"=w586:T1)  [unwired: 6 in, 1 out]
      n141 = property class="ColRmp"(reference=w584, error in=w577, "UnitLabel.Font"=w586, "UnitLabel.Justify"=w585) -> ()  [unwired: 2 out]
    }
    frame "Digital" {
      w608 = refnum<vi> refnum  # Digital
      n142 = To More Specific Class(target class=w608, reference=w610, error in=w609) -> (specific class reference=w600:refnum<vi>)  [unwired: 1 out]
      n143 = call "Variant to Font Data.vi"("Font Key Name"="DigitalNumTextFont", "Fonts LUT in"=w607) -> ("error out"=w597:errorcluster, "Justification"=w598:enum16{"Left", "Center", "Right"}, "Font"=w599:T1, "Fonts LUT out"=w606:variant)  [unwired: 6 in]
      n144 = property class="DigNum"(reference=w600, error in=w597, "NumText.Font"=w599, "NumText.Justify"=w598) -> (reference out=w601:refnum<vi>)  [unwired: 1 out]
      n145 = call "Variant to Font Data.vi"("Font Key Name"="DigitalUnitLabelFont", "Fonts LUT in"=w606) -> ("error out"=w596:errorcluster, "Justification"=w602:enum16{"Left", "Center", "Right"}, "Font"=w603:T1)  [unwired: 6 in, 1 out]
      n146 = property class="DigNum"(reference=w601, error in=w596, "UnitLabel.Font"=w603, "UnitLabel.Justify"=w602) -> ()  [unwired: 2 out]
    }
    frame "NamedNumeric" {
      w629 = refnum<vi> refnum  # NamedNumeric
      n147 = To More Specific Class(target class=w629, reference=w631, error in=w630) -> (specific class reference=w618:refnum<vi>)  [unwired: 1 out]
      n148 = call "Variant to Font Data.vi"("Font Key Name"="NamedNumericRingTextFont", "Fonts LUT in"=w628) -> ("error out"=w617:errorcluster, "Justification"=w615:enum16{"Left", "Center", "Right"}, "Font"=w616:T1, "Fonts LUT out"=w627:variant)  [unwired: 6 in]
      n149 = property class="NmdNum"(reference=w618, error in=w617, "RingText.Font"=w616, "RingText.Justify"=w615) -> (reference out=w619:refnum<vi>)  [unwired: 1 out]
      n150 = call "Variant to Font Data.vi"("Font Key Name"="NamedNumericDigDispFont", "Fonts LUT in"=w627) -> ("error out"=w613:errorcluster, "Justification"=w611:enum16{"Left", "Center", "Right"}, "Font"=w612:T1, "Fonts LUT out"=w626:variant)  [unwired: 6 in]
      n151 = property class="NmdNum"(reference=w619, error in=w613, "DigDisp.Font"=w612, "DigDisp.Justify"=w611) -> (reference out=w620:refnum<vi>)  [unwired: 1 out]
      n152 = call "Variant to Font Data.vi"("Font Key Name"="NamedNumericUnitLabelFont", "Fonts LUT in"=w626) -> ("error out"=w614:errorcluster, "Justification"=w621:enum16{"Left", "Center", "Right"}, "Font"=w622:T1)  [unwired: 6 in, 1 out]
      n153 = property class="NmdNum"(reference=w620, error in=w614, "UnitLabel.Font"=w622, "UnitLabel.Justify"=w621) -> ()  [unwired: 2 out]
    }
    frame "Enum" {
      w650 = refnum<vi> refnum  # Enum
      n154 = To More Specific Class(target class=w650, reference=w652, error in=w651) -> (specific class reference=w639:refnum<vi>)  [unwired: 1 out]
      n155 = call "Variant to Font Data.vi"("Font Key Name"="EnumRingTextFont", "Fonts LUT in"=w649) -> ("error out"=w638:errorcluster, "Justification"=w636:enum16{"Left", "Center", "Right"}, "Font"=w637:T1, "Fonts LUT out"=w648:variant)  [unwired: 6 in]
      n156 = property class="Enum"(reference=w639, error in=w638, "RingText.Font"=w637, "RingText.Justify"=w636) -> (reference out=w640:refnum<vi>)  [unwired: 1 out]
      n157 = call "Variant to Font Data.vi"("Font Key Name"="EnumDigDispFont", "Fonts LUT in"=w648) -> ("error out"=w634:errorcluster, "Justification"=w632:enum16{"Left", "Center", "Right"}, "Font"=w633:T1, "Fonts LUT out"=w647:variant)  [unwired: 6 in]
      n158 = property class="Enum"(reference=w640, error in=w634, "DigDisp.Font"=w633, "DigDisp.Justify"=w632) -> (reference out=w641:refnum<vi>)  [unwired: 1 out]
      n159 = call "Variant to Font Data.vi"("Font Key Name"="EnumUnitLabelFont", "Fonts LUT in"=w647) -> ("error out"=w635:errorcluster, "Justification"=w642:enum16{"Left", "Center", "Right"}, "Font"=w643:T1)  [unwired: 6 in, 1 out]
      n160 = property class="Enum"(reference=w641, error in=w635, "UnitLabel.Font"=w643, "UnitLabel.Justify"=w642) -> ()  [unwired: 2 out]
    }
    frame "Ring" {
      w671 = refnum<vi> refnum  # Ring
      n161 = To More Specific Class(target class=w671, reference=w673, error in=w672) -> (specific class reference=w660:refnum<vi>)  [unwired: 1 out]
      n162 = call "Variant to Font Data.vi"("Font Key Name"="RingRingTextFont", "Fonts LUT in"=w670) -> ("error out"=w659:errorcluster, "Justification"=w657:enum16{"Left", "Center", "Right"}, "Font"=w658:T1, "Fonts LUT out"=w669:variant)  [unwired: 6 in]
      n163 = property class="Ring"(reference=w660, error in=w659, "RingText.Font"=w658, "RingText.Justify"=w657) -> (reference out=w661:refnum<vi>)  [unwired: 1 out]
      n164 = call "Variant to Font Data.vi"("Font Key Name"="RingDigDispFont", "Fonts LUT in"=w669) -> ("error out"=w655:errorcluster, "Justification"=w653:enum16{"Left", "Center", "Right"}, "Font"=w654:T1, "Fonts LUT out"=w668:variant)  [unwired: 6 in]
      n165 = property class="Ring"(reference=w661, error in=w655, "DigDisp.Font"=w654, "DigDisp.Justify"=w653) -> (reference out=w662:refnum<vi>)  [unwired: 1 out]
      n166 = call "Variant to Font Data.vi"("Font Key Name"="RingUnitLabelFont", "Fonts LUT in"=w668) -> ("error out"=w656:errorcluster, "Justification"=w663:enum16{"Left", "Center", "Right"}, "Font"=w664:T1)  [unwired: 6 in, 1 out]
      n167 = property class="Ring"(reference=w662, error in=w656, "UnitLabel.Font"=w664, "UnitLabel.Justify"=w663) -> ()  [unwired: 2 out]
    }
    frame "NumericWithScale" {
      w681 = refnum<vi> refnum  # NumericWithScale
      n168 = To More Specific Class(target class=w681, reference=w684, error in=w683) -> (specific class reference=w682:refnum<vi>, error out=w677:errorcluster)
      n169 = call "Variant to Font Data.vi"("error in"=w677, "Font Key Name"="NumericWithScaleUnitLabelFont", "Fonts LUT in"=w679) -> ("error out"=w676:errorcluster, "Justification"=w674:enum16{"Left", "Center", "Right"}, "Font"=w675:T1)  [unwired: 5 in, 1 out]
      n170 = property class="NumWthScl"(reference=w682, error in=w676, "UnitLabel.Font"=w675, "UnitLabel.Justify"=w674) -> (error out=w680:errorcluster)  [unwired: 1 out]
    }
    frame "Knob" {
      w699 = refnum<vi> refnum  # Knob
      n171 = To More Specific Class(target class=w699, reference=w701, error in=w700) -> (specific class reference=w689:refnum<vi>, error out=w692:errorcluster)
      n172 = call "Variant to Font Data.vi"("error in"=w692, "Font Key Name"="KnobMarkerFont", "Fonts LUT in"=w698) -> ("error out"=w685:errorcluster, "Justification"=w686:enum16{"Left", "Center", "Right"}, "Font"=w687:T1, "Fonts LUT out"=w697:variant)  [unwired: 5 in]
      n173 = property class="Knob"(reference=w689, error in=w685, "Active Slider"=0, "Scale.Marker.Font"=w687, "Scale.Marker.Justify"=w686) -> (reference out=w688:refnum<vi>)  [unwired: 1 out]
      n174 = call "Variant to Font Data.vi"("Font Key Name"="KnobUnitLabelFont", "Fonts LUT in"=w697) -> ("error out"=w691:errorcluster, "Justification"=w693:enum16{"Left", "Center", "Right"}, "Font"=w694:T1)  [unwired: 6 in, 1 out]
      n175 = property class="Knob"(reference=w688, error in=w691, "UnitLabel.Font"=w694, "UnitLabel.Justify"=w693) -> ()  [unwired: 2 out]
    }
    frame "Slide" {
      w716 = refnum<vi> refnum  # Slide
      n176 = To More Specific Class(target class=w716, reference=w718, error in=w717) -> (specific class reference=w706:refnum<vi>, error out=w709:errorcluster)
      n177 = call "Variant to Font Data.vi"("error in"=w709, "Font Key Name"="SlideScaleMarkerFont", "Fonts LUT in"=w715) -> ("error out"=w702:errorcluster, "Justification"=w703:enum16{"Left", "Center", "Right"}, "Font"=w704:T1, "Fonts LUT out"=w714:variant)  [unwired: 5 in]
      n178 = property class="Slide"(reference=w706, error in=w702, "Active Slider"=0, "Scale.Marker.Font"=w704, "Scale.Marker.Justify"=w703) -> (reference out=w705:refnum<vi>)  [unwired: 1 out]
      n179 = call "Variant to Font Data.vi"("Font Key Name"="SlideUnitLabelFont", "Fonts LUT in"=w714) -> ("error out"=w708:errorcluster, "Justification"=w710:enum16{"Left", "Center", "Right"}, "Font"=w711:T1)  [unwired: 6 in, 1 out]
      n180 = property class="Slide"(reference=w705, error in=w708, "UnitLabel.Font"=w711, "UnitLabel.Justify"=w710) -> ()  [unwired: 2 out]
    }
    frame "Path" {
      w726 = refnum<vi> refnum  # Path
      n181 = To More Specific Class(target class=w726, reference=w729, error in=w728) -> (specific class reference=w727:refnum<vi>, error out=w720:errorcluster)
      n182 = call "Variant to Font Data.vi"("error in"=w720, "Font Key Name"="PathTextFont", "Fonts LUT in"=w725) -> ("error out"=w721:errorcluster, "Justification"=w722:enum16{"Left", "Center", "Right"}, "Font"=w723:T1)  [unwired: 5 in, 1 out]
      n183 = property class="Path"(reference=w727, error in=w721, "Text.Font"=w723, "Text.Justify"=w722) -> (error out=w719:errorcluster)  [unwired: 1 out]
    }
    frame "String" {
      w737 = refnum<vi> refnum  # String
      n184 = To More Specific Class(target class=w737, reference=w740, error in=w739) -> (specific class reference=w738:refnum<vi>, error out=w733:errorcluster)
      n185 = call "Variant to Font Data.vi"("error in"=w733, "Font Key Name"="StringTextFont", "Fonts LUT in"=w735) -> ("error out"=w732:errorcluster, "Justification"=w730:enum16{"Left", "Center", "Right"}, "Font"=w731:T1)  [unwired: 5 in, 1 out]
      n186 = property class="Str"(reference=w738, error in=w732, "Text.Font"=w731, "Text.Justify"=w730) -> (error out=w736:errorcluster)  [unwired: 1 out]
    }
    frame "ComboBox" {
      w748 = refnum<vi> refnum  # ComboBox
      n187 = To More Specific Class(target class=w748, reference=w751, error in=w750) -> (specific class reference=w749:refnum<vi>, error out=w744:errorcluster)
      n188 = call "Variant to Font Data.vi"("error in"=w744, "Font Key Name"="ComboBoxTextFont", "Fonts LUT in"=w746) -> ("error out"=w743:errorcluster, "Justification"=w741:enum16{"Left", "Center", "Right"}, "Font"=w742:T1)  [unwired: 5 in, 1 out]
      n189 = property class="CmbBox"(reference=w749, error in=w743, "Text.Font"=w742, "Text.Justify"=w741) -> (error out=w747:errorcluster)  [unwired: 1 out]
    }
    frame "Table" {
      w760 = refnum<vi> refnum  # Table
      n190 = To More Specific Class(target class=w760, reference=w763, error in=w762) -> (specific class reference=w761:refnum<vi>, error out=w755:errorcluster)
      n191 = call "Variant to Font Data.vi"("error in"=w755, "Font Key Name"="TableActiveCellFont", "Fonts LUT in"=w757) -> ("error out"=w754:errorcluster, "Justification"=w752:enum16{"Left", "Center", "Right"}, "Font"=w753:T1)  [unwired: 5 in, 1 out]
      n192 = property class="Tbl"(reference=w761, error in=w754, "Active Cell"=T2 {"Row"=-2, "Column"=-2} ("Active Cell:Active Cell"), "CellFont"=w753, "Justify"=w752) -> (error out=w759:errorcluster)  [unwired: 1 out]
    }
    frame "TreeControl" {
      w772 = refnum<vi> refnum  # TreeControl
      n193 = To More Specific Class(target class=w772, reference=w775, error in=w774) -> (specific class reference=w773:refnum<vi>, error out=w768:errorcluster)
      n194 = call "Variant to Font Data.vi"("error in"=w768, "Font Key Name"="TreeControlActiveColFont", "Fonts LUT in"=w770) -> ("error out"=w767:errorcluster, "Justification"=w765:enum16{"Left", "Center", "Right"}, "Font"=w766:T1)  [unwired: 5 in, 1 out]
      n195 = property class="Tree"(reference=w773, error in=w767, "ActiveColNum"=-2 ("Active Cell:Active Column Number"), "CellFont"=w766, "Justify"=w765) -> (error out=w771:errorcluster)  [unwired: 1 out]
    }
  }
  "Error Out" <- w1
  "FontUIP Out" <- "FontUIP In"
